vi "Practica5.vi"() -> ()   [LabVIEW 2024]
panel:
  out "Indicador":string
  out "V/F":bool
  out "Segundos":dbl
  out "Minutos":dbl
  out "Horas":dbl
  in  "Tiempo en segundos":dbl
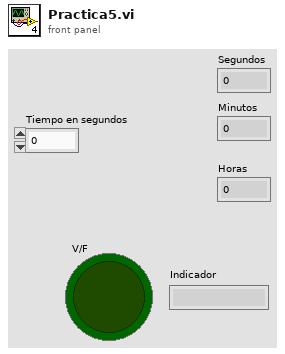
[diagram p1: front panel]
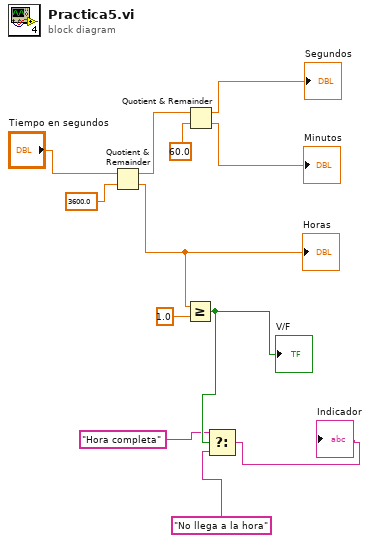
[diagram p0: block diagram]
diagram:
  n1 = Quotient & Remainder(x="Tiempo en segundos", y=3600.0 ("floor(x/y)")) -> (x-y*floor(x/y)=w10:dbl, floor(x/y)=w5:dbl)
  "Horas" <- w5
  n2 = Greater Or Equal?(x=w5, y=1.0) -> (x >= y?=w4:bool)
  "V/F" <- w4
  n3 = Quotient & Remainder(x=w10, y=60.0 ("x-y*floor(x/y)")) -> (x-y*floor(x/y)=→"Segundos":dbl, floor(x/y)=→"Minutos":dbl)
  n4 = Select(t="Hora completa" ("Indicador"), s=w4, f="No llega a la hora" ("Indicador")) -> (s? t:f=→"Indicador":string)
